vi "Get Last Values.vi"(8 "error in (no error)":errorcluster, 10 "Variables":string[](array[string]), 11 "Output Sequencer in":refnum<class "Output Sequencer.lvclass">) -> (0 "error out":errorcluster, 2 "Values":dbl[](array[numeric]), 3 "Output Sequencer out":refnum<class "Output Sequencer.lvclass">)   [LabVIEW 2020, in "Output Sequencer.lvlib" / "Output Sequencer.lvclass"]
uses:
  Output Sequencer.lvclass
  Output Sequencer.lvclass/Output Sequencer.ctl
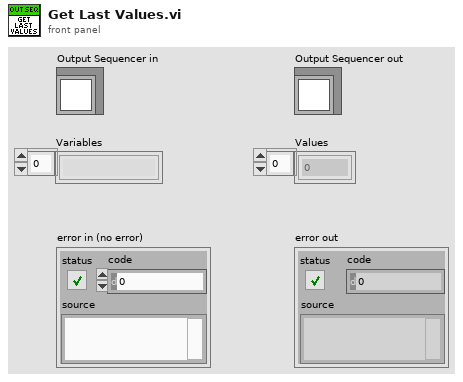
[diagram p1: front panel]
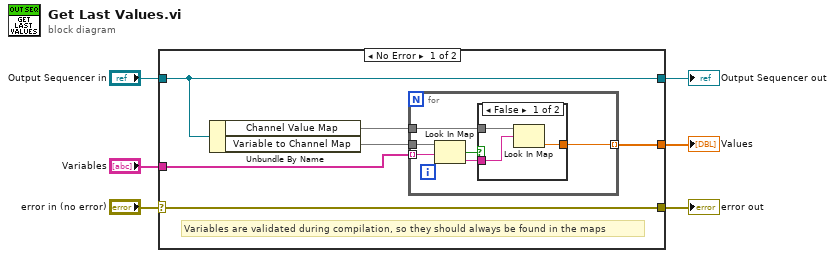
[diagram p0: block diagram]
diagram:
  n1 = case shown="No Error" "error in (no error)" {
    selector: "error in (no error)" -> [w8 w22]
    tunnel: "Output Sequencer in" -> [w7 w23]
    tunnel: [w12 _] -> w5
    tunnel: "Variables" -> [w11 _]
    tunnel: [w8 w22] -> w2
    tunnel: [w7 w23] -> w1
    frame No Error {
      # "Variables are validated during compilation, so they should always be found in the maps"
      n2 = Unbundle By Name(w7) -> ("Channel Value Map"=w10:map{string, dbl}, "Variable to Channel Map"=w9:map{string, string})
      n3 = for {
        tunnel: [w18] -> w12 mode=indexing
        tunnel: w11 -> [w15] mode=indexing
        tunnel: w10 -> [w17]
        tunnel: w9 -> [w16]
        n4 = Look In Map(map=w16, key=w15) -> (key not found?=w13:bool, value=w14:string)  [unwired: 1 in]
        n5 = case shown="False" w13 {
          tunnel: [w21 _] -> w18
          tunnel: w17 -> [w20 _]
          tunnel: w14 -> [w19 _]
          frame False {
            n6 = Look In Map(map=w20, key=w19) -> (value=w21:dbl)  [unwired: 1 in, 1 out]
          }
          frame True {
          }
        }
      }
    }
    frame Error {
    }
  }
  "Output Sequencer out" <- w1
  "Values" <- w5
  "error out" <- w2
